vi "DrawSnake.vi"(8 "error in (no error)":errorcluster, 10 "SnakeData":T1, 11 "Snake in":refnum<class "SnakeGame.lvclass">) -> (0 "error out":errorcluster, 3 "Snake out":refnum<class "SnakeGame.lvclass">)   [LabVIEW 2019, in "RT_Game.lvlib" / "SnakeGame.lvclass"]
uses:
  SnakeGame.lvclass
  C:/Users/FreshBob/Dropbox/VIs/myRIO_GameConsole/RT/RT_Game/Game/Game.lvclass
  SnakeData.ctl
  Direction.ctl
  Game/Coordinate.ctl
  CoordinateData.ctl
  Game/Game.lvclass
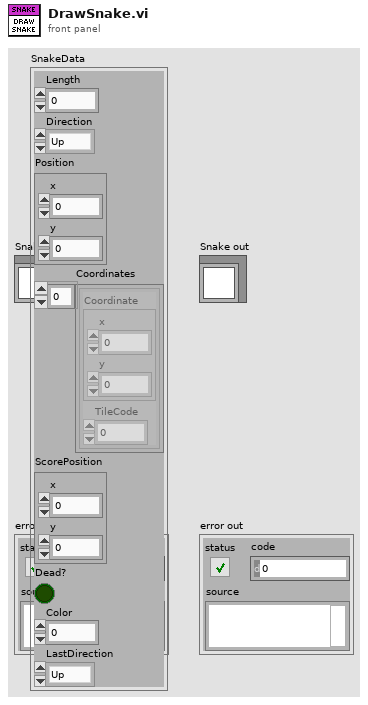
[diagram p1: front panel]
types:
  T1 = typedef "RT_Game.lvlib/SnakeGame.lvclass/SnakeData.ctl" = cluster{"Length":i16, "Direction":T2, "Position":T3, "Coordinates":T4[], "ScorePosition":T3, "Dead?":bool, "Color":fxp<+,3,3>, "LastDirection":T2}
  T2 = typedef "RT_Game.lvlib/SnakeGame.lvclass/Direction.ctl" = enum16{"Up", "Left", "Down", "Right"}
  T3 = typedef "RT_Game.lvlib/Game.lvclass/Coordinate.ctl" = cluster{"x":dbl, "y":dbl}
  T4 = typedef "RT_Game.lvlib/SnakeGame.lvclass/CoordinateData.ctl" = cluster{"Coordinate":T3, "TileCode":u16}
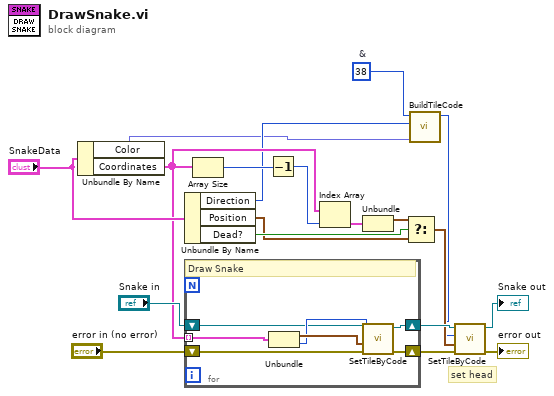
[diagram p0: block diagram]
diagram:
  w4 = u16 38  # &
  # "set head"
  n1 = Unbundle By Name("SnakeData") -> ("Color"=w2:fxp<+,3,3>, "Coordinates"=w11:T4[])
  n2 = Unbundle By Name("SnakeData") -> ("Direction"=w3:T2, "Position"=w6:T3, "Dead?"=w8:bool)
  n3 = for {
    shift-right: [w25] -> w16
    shift-left: "error in (no error)" -> [w26]
    shift-right: [w24] -> w17
    shift-left: "Snake in" -> [w20]
    tunnel: w11 -> [w23] mode=indexing
    # "Draw Snake"
    n4 = Unbundle(w23) -> ("Coordinate"=w22:T3, "TileCode"=w21:u16)
    n5 = call "SetTileByCode.vi"("error in (no error)"=w26, "Coordinates"=w22, "TileNumber"=w21, "Game in"=w20) -> ("error out"=w25:errorcluster, "Game out"=w24:refnum<class "SnakeGame.lvclass">)  [unwired: 6 in]
  }
  n6 = Array Size(array=w11) -> (size(s)=w10:i32)
  n7 = Decrement(x=w10) -> (x-1=w9:i32)
  n8 = Index Array(array=w11, index=w9) -> (element=w7:T4)
  n9 = Unbundle(w7) -> ("Coordinate"=w5:T3)  [unwired: 1 out]
  n10 = Select(t=w5, s=w8, f=w6) -> (s? t:f=w12:T3)
  n11 = call "BuildTileCode.vi"("replace_color"=w2, "rotation"=w3, "tilenumber"=w4) -> ("TileCode"=w1:u16)  [unwired: 8 in]
  n12 = call "SetTileByCode.vi"("error in (no error)"=w16, "Coordinates"=w12, "TileNumber"=w1, "Game in"=w17) -> ("error out"=→"error out":errorcluster, "Game out"=→"Snake out":refnum<class "SnakeGame.lvclass">)  [unwired: 6 in]
